vi "random values.vi"() -> ()   [LabVIEW 2016]
panel:
  in  "stop":bool
  out "Waveform Chart":dbl(graph)
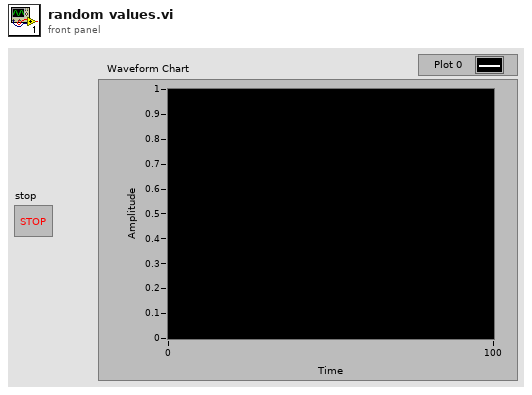
[diagram p1: front panel]
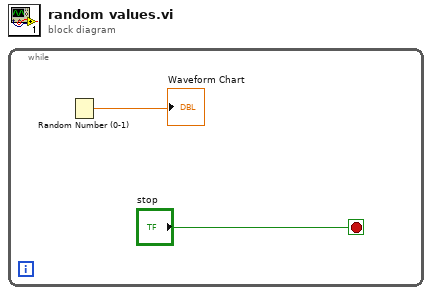
[diagram p0: block diagram]
diagram:
  n1 = while {
    stop <- "stop" stop-if-true
    n2 = Random Number (0-1)() -> (number: 0 to 1=→"Waveform Chart":dbl)
  }
